vi "Wait (ms) with error IO.vi"(3 "error in (no error)":errorcluster, 4 "milliseconds to wait":u32) -> (0 "error out":errorcluster)   [LabVIEW 2013, in "Timing Lib.lvlib"]
doc: "Same as labview vi \"wait (ms)\" except that error IO has been added."
uses:
  Timing Lib.lvlib
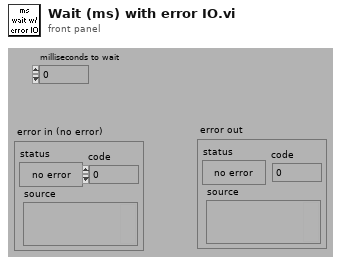
[diagram p1: front panel]
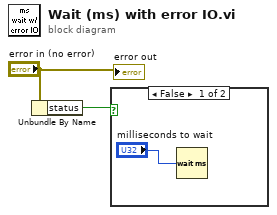
[diagram p0: block diagram]
diagram:
  n1 = Unbundle By Name("error in (no error)") -> ("status"=w1:bool)
  n2 = case shown="False" w1 {
    frame False {
      n3 = Wait (ms)(milliseconds to wait="milliseconds to wait") -> ()  [unwired: 1 out]
    }
    frame True {
    }
  }
  "error out" <- "error in (no error)"
